vi "GPS on GIC 4.vi"(1 "GIC Input":T1={"Real/Sim"=FALSE, "WP Lats and Longs"={"WP Lats"=[], "WP Longs"=[]}, "GPS Time Int"=0.0, "GPS Com Port"="", "Compass Com Port"="", "Prop Com Port"="", "GPS Data"=[], "Compass"=0.0, "LMS Vector"=[], "Vision Vector"=[], "Direction Cmd"=0.0, "Speed Cmd"=0.0, "Time of Last GPS"=0.0, "WP Vector"=[], "WP Number"=0, "Num of WPs"=0, "SW Map"=[], "Obst Lats and Longs"={"Obst Lats"=[], "Obst Longs"=[]}, "Parameters"=[], "Path Cluster"={"Path x nodes"=[], "Path y nodes"=[]}, "     Use ?\nOff       On"=[TRUE, TRUE, FALSE, FALSE]} {"Obst Lats and Longs"."Obst Longs" format="%#_8g"; "Obst Lats and Longs"."Obst Lats" format="%#_8g"}) -> (0 "GIC Output":T1={"Real/Sim"=FALSE, "WP Lats and Longs"={"WP Lats"=[], "WP Longs"=[]}, "GPS Time Int"=0.0, "GPS Com Port"="", "Compass Com Port"="", "Prop Com Port"="", "GPS Data"=[], "Compass"=0.0, "LMS Vector"=[], "Vision Vector"=[], "Direction Cmd"=0.0, "Speed Cmd"=0.0, "Time of Last GPS"=0.0, "WP Vector"=[], "WP Number"=0, "Num of WPs"=0, "SW Map"=[], "Obst Lats and Longs"={"Obst Lats"=[], "Obst Longs"=[]}, "Parameters"=[], "Path Cluster"={"Path x nodes"=[], "Path y nodes"=[]}, "     Use ?\nOff       On"=[TRUE, TRUE, FALSE, FALSE]} {"Obst Lats and Longs"."Obst Longs" format="%#_8g"; "Obst Lats and Longs"."Obst Lats" format="%#_8g"})   [LabVIEW 2014]
panel:
  # "GPS"
  # "LMS"
  # "Vision"
  # "Prop"
  # "GPS"
  # "LMS"
  # "Vision"
  # "Prop"
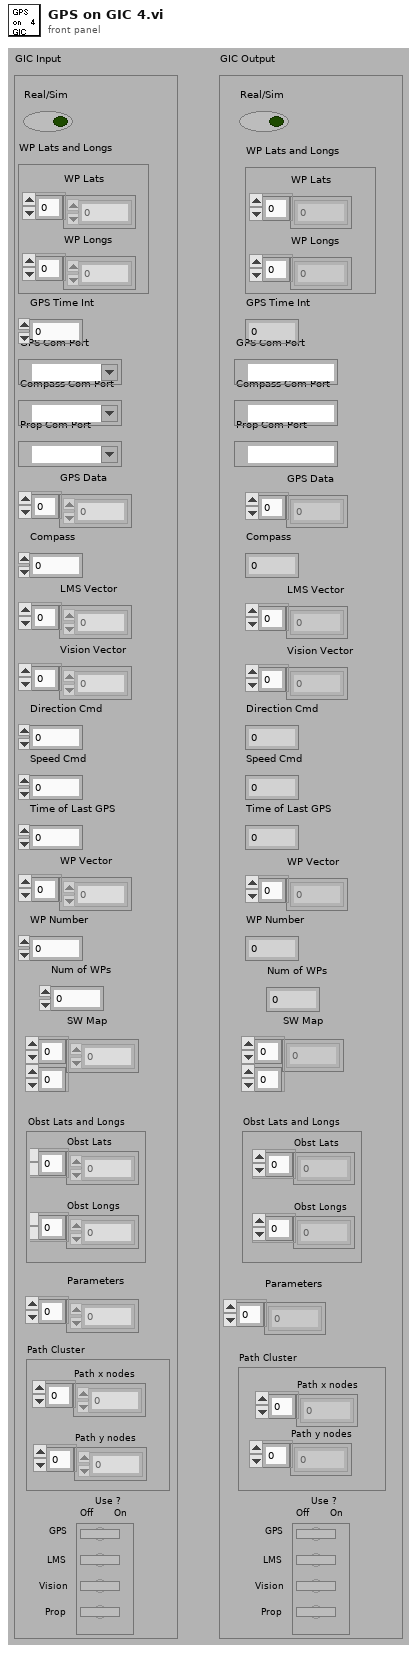
[diagram p1: front panel]
types:
  T1 = cluster{"Real/Sim":bool, "WP Lats and Longs":cluster{"WP Lats":dbl[], "WP Longs":dbl[]}, "GPS Time Int":dbl, "GPS Com Port":refnum<visa-resource-name>, "Compass Com Port":refnum<visa-resource-name>, "Prop Com Port":refnum<visa-resource-name>, "GPS Data":dbl[], "Compass":dbl, "LMS Vector":dbl[], "Vision Vector":dbl[], "Direction Cmd":dbl, "Speed Cmd":dbl, "Time of Last GPS":dbl, "WP Vector":dbl[], "WP Number":i32, "Num of WPs":i16, "SW Map":i32[][], "Obst Lats and Longs":cluster{"Obst Lats":dbl[], "Obst Longs":dbl[]}, "Parameters":dbl[], "Path Cluster":cluster{"Path x nodes":dbl[], "Path y nodes":dbl[]}, "     Use ?\nOff       On":bool[]}
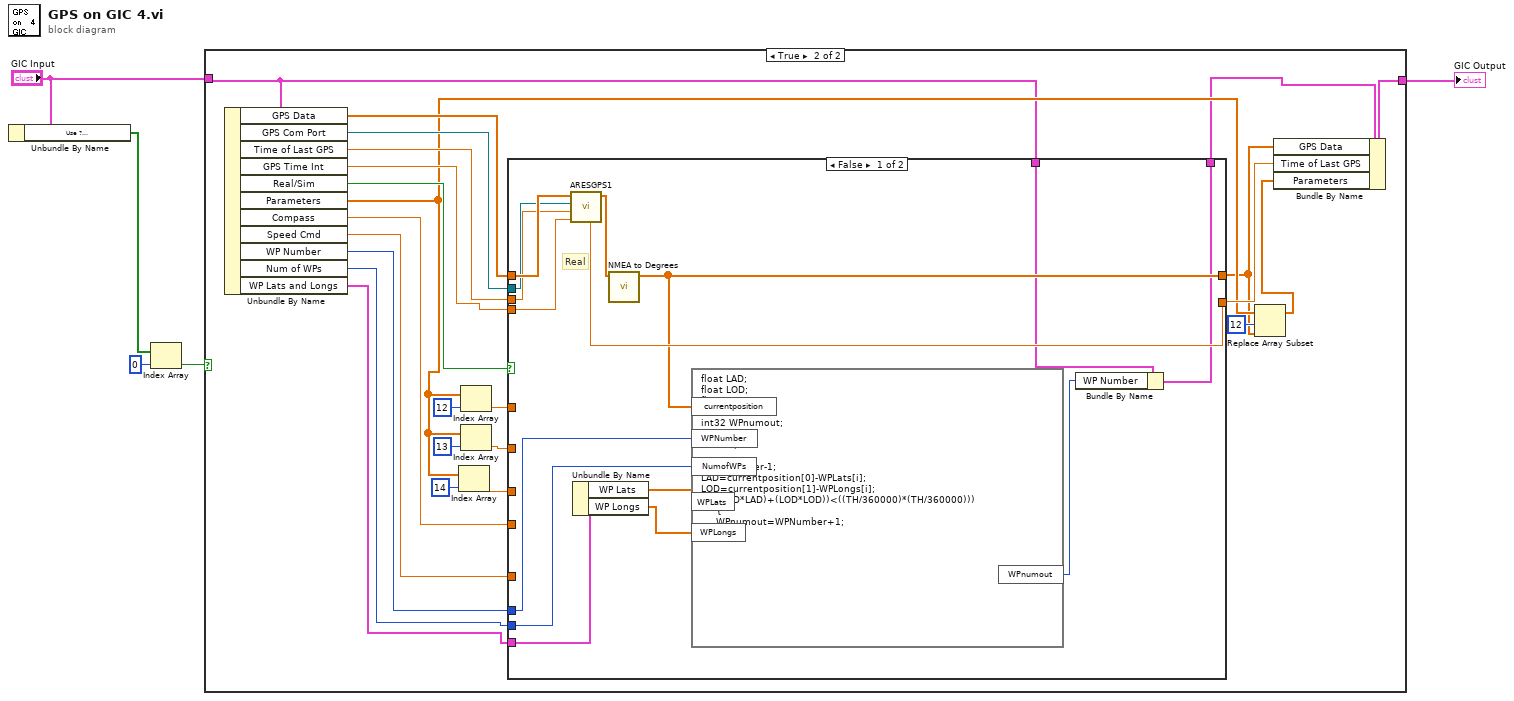
[diagram p0: block diagram]
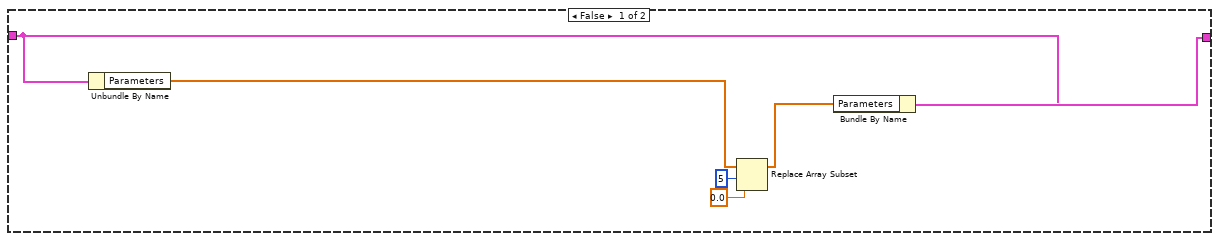
[diagram p2: hidden frame]
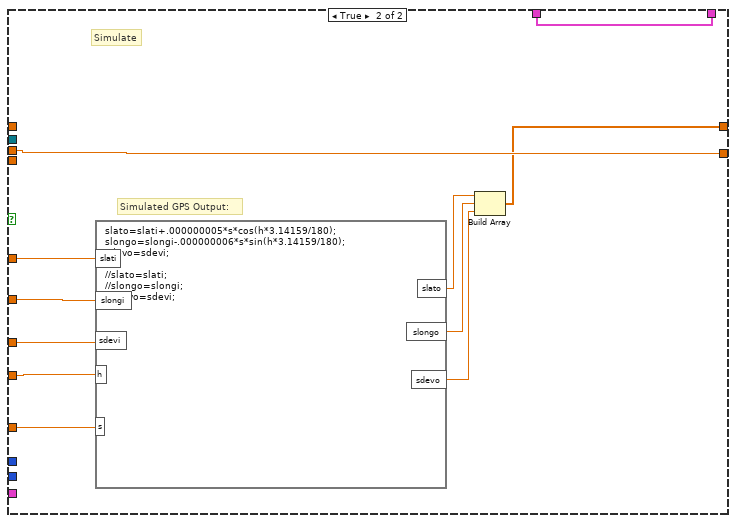
[diagram p3: hidden frame]
diagram:
  n1 = Unbundle By Name("GIC Input") -> ("Use ?\nOff       On"=w3:bool[])
  n2 = Index Array(array=w3, index=0) -> (element=w1:bool)
  n3 = case shown="True" w1 {
    tunnel: "GIC Input" -> [w6 w13]
    tunnel: [w11 w17] -> w5
    frame False {
      n4 = Unbundle By Name(w6) -> ("Parameters"=w10:dbl[])
      n5 = Replace Array Subset(array=w10, new element=0.0 ("new element/subarray"), index=5) -> (w8:dbl[])
      n6 = Bundle By Name(cluster=w6, "Parameters"=w8) -> (w11:T1)
    }
    frame True {
      n7 = Unbundle By Name(w13) -> ("GPS Data"=w30:dbl[], "GPS Com Port"=w31:refnum<visa-resource-name>, "Time of Last GPS"=w32:dbl, "GPS Time Int"=w33:dbl, "Real/Sim"=w34:bool, "Parameters"=w23:dbl[], "Compass"=w19:dbl, "Speed Cmd"=w18:dbl, "WP Number"=w16:i32, "Num of WPs"=w15:i16, "WP Lats and Longs"=w14:cluster{"WP Lats":dbl[], "WP Longs":dbl[]})
      n8 = Index Array(array=w23, index=14) -> (element=w24:dbl)
      n9 = Index Array(array=w23, index=12) -> (element=w26:dbl)
      n10 = Index Array(array=w23, index=13) -> (element=w25:dbl)
      n11 = case shown="False" w34 {
        tunnel: w30 -> [w50 _]
        tunnel: [w44 w54] -> w21
        tunnel: w31 -> [w49 _]
        tunnel: w32 -> [w48 w61]
        tunnel: w33 -> [w47 _]
        tunnel: [w46 w61] -> w35
        tunnel: w26 -> [_ w60]
        tunnel: w25 -> [_ w59]
        tunnel: w24 -> [_ w58]
        tunnel: w19 -> [_ w53]
        tunnel: w18 -> [_ w52]
        tunnel: w16 -> [w43 _]
        tunnel: w15 -> [w42 _]
        tunnel: w14 -> [w41 _]
        tunnel: w13 -> [w38 w51]
        tunnel: [w37 w51] -> w12
        frame False {
          # "Real"
          n12 = call "ARESGPS1.vi"("GPS Time interval Input"=w47, "Input time of last gps read"=w48, "GPS Com Port"=w49, "Input lat, long, dev"=w50) -> ("Output lat, long, dev"=w45:dbl[], "Output time of last GPS read"=w46:dbl)  [unwired: 3 in, 3 out]
          n13 = Unbundle By Name(w41) -> ("WP Lats"=w40:dbl[], "WP Longs"=w39:dbl[])
          n14 = call "NMEA to Degrees.vi"("NMEA Input"=w45) -> ("Degrees Output"=w44:dbl[])  [unwired: 10 in]
          n15 = formula code="float LAD;\nfloat LOD;\nfloat TH;\nint i;\nint32 WPnumout;\n\nTH=10;\n\ni=WPNumber-1;\nLAD=currentposition[0]-WPLats[i];\nLOD=currentposition[1]-WPLongs[i];\nif (((LAD*LAD)+(LOD*LOD))<((TH/360000)*(TH/360000)))\n     {\n     WPnumout=WPNumber+1;\n     }"("currentposition"=w44, "WPNumber"=w43, "NumofWPs"=w42, "WPLats"=w40, "WPLongs"=w39) -> ("WPnumout"=w36:i32)
          n16 = Bundle By Name(cluster=w38, "WP Number"=w36) -> (w37:T1)
        }
        frame True {
          # "Simulated GPS Output:"
          # "Simulate"
          n17 = formula code="slato=slati+.000000005*s*cos(h*3.14159/180);\nslongo=slongi-.000000006*s*sin(h*3.14159/180);\nsdevo=sdevi;\n\n//slato=slati;\n//slongo=slongi;\n//sdevo=sdevi;"("slati"=w60, "slongi"=w59, "sdevi"=w58, "h"=w53, "s"=w52) -> ("slato"=w57:dbl, "slongo"=w56:dbl, "sdevo"=w55:dbl)
          n18 = Build Array(w57, w56, w55) -> (w54:dbl[])
        }
      }
      n19 = Replace Array Subset(array=w23, new element=w21, index=12) -> (w20:dbl[])
      n20 = Bundle By Name(cluster=w12, "GPS Data"=w21, "Time of Last GPS"=w35, "Parameters"=w20) -> (w17:T1)
    }
  }
  "GIC Output" <- w5
